vi "From Veristand Master To Modbus.vi"(7 "Parameters":T1 {"Interface Data"."Serial Settings"."parity (even)" items=["None", "Odd", "Even", "Mark", "Space"]; "Interface Data"."Serial Settings"."flow control (none)" items=["None", "XON/XOFF", "RTS/CTS", "XON/XOFF & RTS/CTS", "DTR/DSR", "XON/XOFF & DTR/DSR"]}, 8 "error in (no error)":errorcluster, 10 "Process in":refnum<class "Process.lvclass">, 11 "Modbus Master in":refnum<class "Modbus Master.lvclass">) -> ()   [LabVIEW 2015, in "Modbus Master Engine.lvlib"]
uses:
  Modbus Master Engine.lvlib
  <vilib>/addons/Inline Async API/_VS Inline Async API/Process/Process.lvclass
  Shared/Device Info.ctl
  Shared/Controls/Interface Type.ctl
  Shared/Controls/Data Model/TCP Settings.ctl
  Shared/Controls/Data Model/Serial Settings.ctl
  Bulk Data Access.ctl
  System Explorer/SubVIs/Modbus Type.ctl
  Shared/Controls/Data Model/Channel.ctl
  <vilib>/NI Veristand/Custom Device API/Custom Device Channel Type.ctl
  Shared/Controls/Data Model/Mapping.ctl
  Shared/Controls/Data Model/DataType.ctl
  <vilib>/NI Veristand/Custom Device API/Custom Device Item Ref.ctl
  Modbus API.lvlibp/API/Master/Modbus Master.lvclass
  <vilib>/addons/Inline Async API/_Data Access Engine/Access Type Classes/Read/Read.lvclass/Read.ctl
  <vilib>/addons/Inline Async API/_VS Inline Async API/Process/Process.lvclass/Process.ctl
  <vilib>/addons/Inline Async API/_Data Access Engine/Access Type Classes/Read/Read.ProcessData.vi
  <vilib>/addons/Inline Async API/_Data Access Engine/Data Access Engine/Methods/Read.Data.vi
  <vilib>/addons/Inline Async API/_Data Access Engine/Data Access Engine/Data Access Engine.lvclass
  Shared/Modbus Master Shared.lvlib
  <vilib>/NI VeriStand/Custom Device API/Custom Device API.lvlib
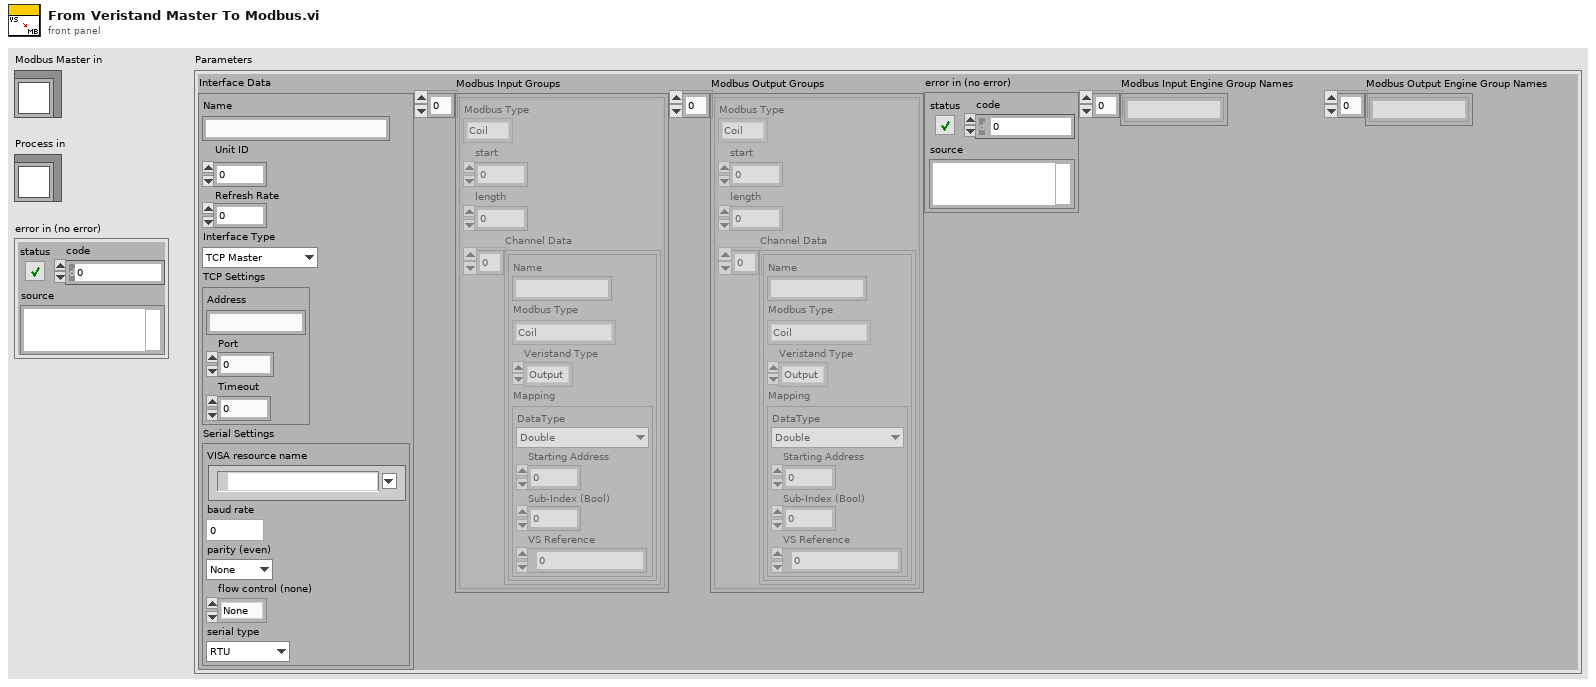
[diagram p1: front panel]
types:
  T1 = typedef "Modbus Master Shared.lvlib/Device Info.ctl" = cluster{"Interface Data":cluster{"Name":string, "Unit ID":u8, "Refresh Rate":i32, "Interface Type":T2, "TCP Settings":T3, "Serial Settings":T4}, "Modbus Input Groups":T5[], "Modbus Output Groups":T5[], "error in (no error)":errorcluster, "Modbus Input Engine Group Names":string[], "Modbus Output Engine Group Names":string[]}
  T2 = typedef "Modbus Master Shared.lvlib/Interface Type.ctl" = enum16{"TCP Master", "Serial Master", "TCP Slave", "Serial Slave"}
  T3 = typedef "Modbus Master Shared.lvlib/TCP Settings.ctl" = cluster{"Address":string, "Port":u16, "Timeout":i32}
  T4 = typedef "Modbus Master Shared.lvlib/Serial Settings.ctl" = cluster{"VISA resource name":refnum<visa-resource-name>, "baud rate":u32, "parity (even)":u16, "flow control (none)":u16, "serial type":enum16{"RTU", "ASCII"}}
  T5 = typedef "Modbus Master Shared.lvlib/Bulk Data Access.ctl" = cluster{"Modbus Type":T6, "start":u16, "length":u16, "Channel Data":T7[]}
  T6 = typedef "Modbus Master Shared.lvlib/Modbus Type.ctl" = enum16{"Coil", "Discrete Input", "Holding Register", "Input Register"}
  T7 = typedef "Modbus Master Shared.lvlib/Channel.ctl" = cluster{"Name":string, "Modbus Type":T6, "Veristand Type":T8, "Mapping":T9}
  T8 = typedef "Custom Device API.lvlib/Custom Device Channel Type.ctl" = enum16{"Input", "Output"}
  T9 = typedef "Modbus Master Shared.lvlib/Mapping.ctl" = cluster{"DataType":T10, "Starting Address":u16, "Sub-Index (Bool)":u16, "VS Reference":T11}
  T10 = typedef "Modbus Master Shared.lvlib/DataType.ctl" = enum16{"Double", "Single", "I64", "I32", "I16", "I8", "U64", "U32", "U16", "U8", "Boolean"}
  T11 = typedef "Custom Device API.lvlib/Custom Device Item Ref.ctl" = u64
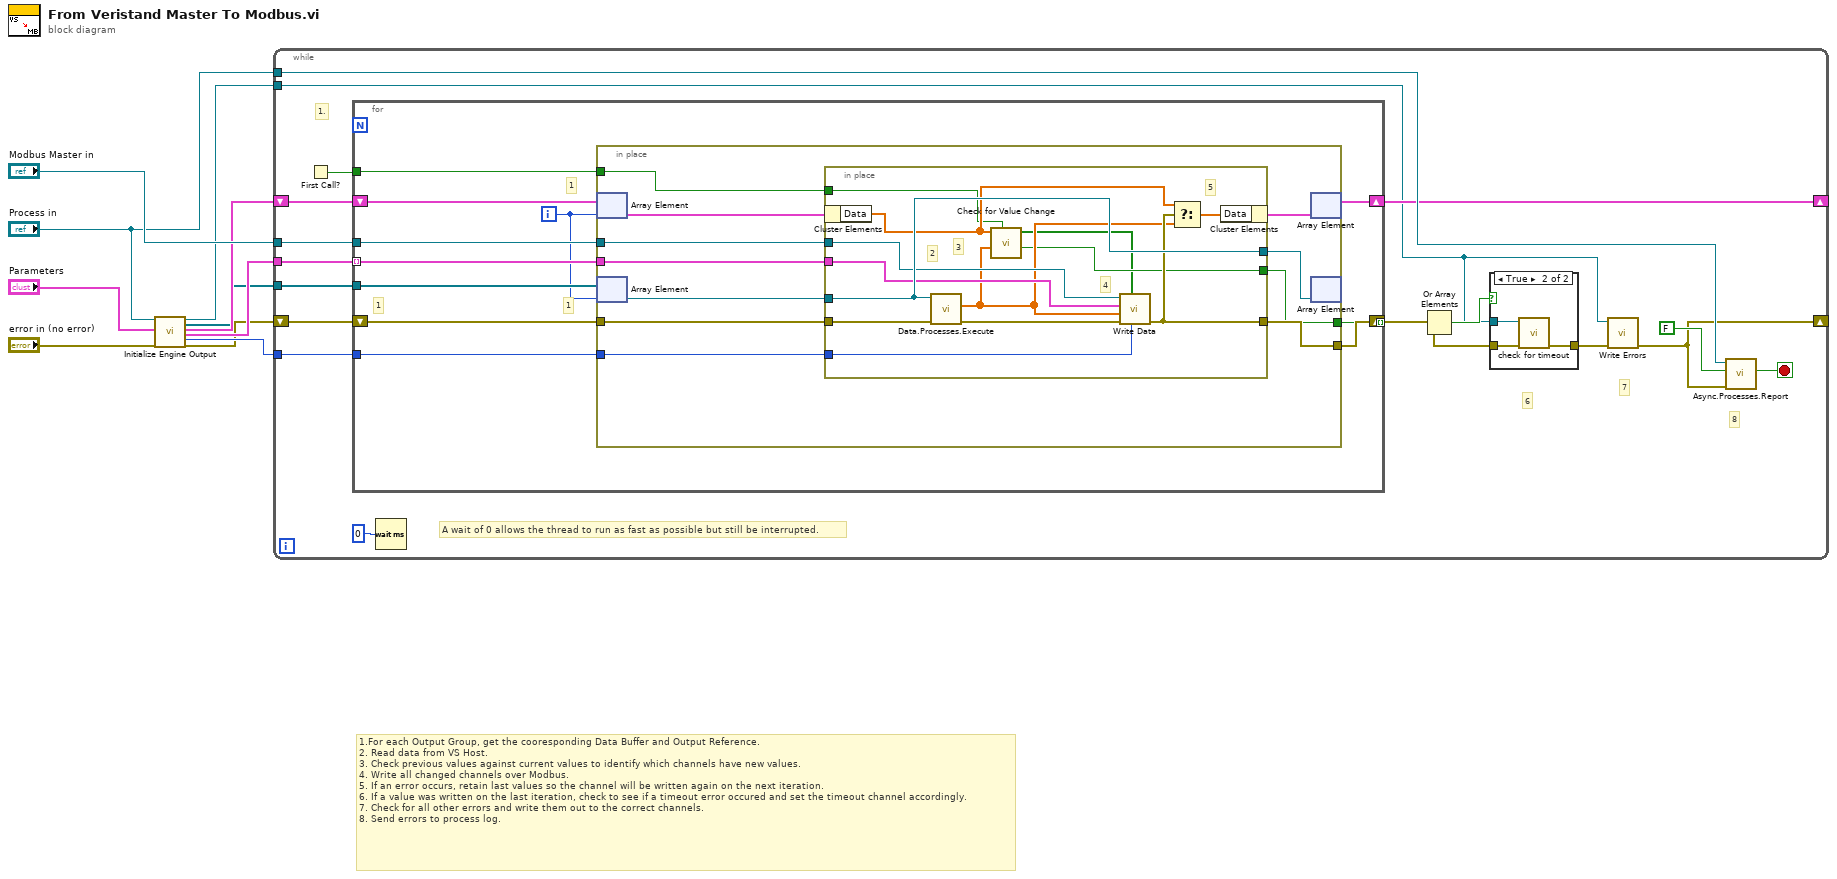
[diagram p0: block diagram]
diagram:
  # "1.For each Output Group, get the cooresponding Data Buffer and Output Reference.\n2. Read data from VS Host.\n3. Check previous values against current values to identify which channels have new values.\n4. Write all changed channels over Modbus.\n5. If an error occurs, retain last values so the channel will be written again on the next iteration.\n6. If a value was written on the last iteration, check to see if a timeout error occured and set the timeout channel accordingly.\n7. Check for all other errors and write them out to the correct channels.\n8. Send errors to process log."
  n1 = call "Initialize Engine Output.vi"("Process in"="Process in", "Parameters"="Parameters", "error in (no error)"="error in (no error)") -> ("Diagnostic Group Ref"=w3:refnum<data-value>, "Output Group Refs"=w5:refnum<data-value>[], "Data Buffers"=w7:cluster{"Data":dbl[]}[], "Modbus Output Groups"=w8:T5[], "Unit ID"=w2:u8, "error out"=w1:errorcluster)  [unwired: 11 in]
  n2 = while {
    tunnel: "Process in" -> [w28]
    tunnel: w5 -> [w25]
    tunnel: w8 -> [w27]
    tunnel: "Modbus Master in" -> [w26]
    shift-right: [w22] -> _
    shift-left: w7 -> [w23]
    tunnel: w3 -> [w11]
    tunnel: w2 -> [w18]
    shift-right: [w17] -> _
    shift-left: w1 -> [w16]
    stop <- w24 stop-if-true
    # "8"
    # "7"
    # "6"
    # "A wait of 0 allows the thread to run as fast as possible but still be interrupted."
    # "1."
    n3 = First Call?() -> (First Call?: T/F=w19:bool)
    n4 = for {
      tunnel: w27 -> [w38] mode=indexing
      tunnel: w26 -> [w39]
      tunnel: w25 -> [w34]
      shift-right: [w35] -> w22
      shift-left: w23 -> [w36]
      tunnel: w19 -> [w32]
      tunnel: w18 -> [w31]
      shift-right: [w30] -> w15
      shift-left: w16 -> [w37]
      tunnel: [w29] -> w13 mode=indexing
      i -> [w33]
      # "1"
      # "1"
      # "1"
      n5 = in-place {
        in-place-border: w39 -> [w50]
        in-place-border: w38 -> [w49]
        in-place-border: w37 -> [w48]
        in-place-border: [w47] -> w30
        in-place-border: w32 -> [w42]
        in-place-border: w31 -> [w41]
        in-place-border: [w40] -> w29
        n6 = in-place-array #1(w36, w33) -> (w46:cluster{"Data":dbl[]})
        n7 = in-place-array #2(w34, w33) -> (w44:refnum<data-value>)
        n8 = in-place {
          in-place-border: w50 -> [w61]
          in-place-border: w49 -> [w58]
          in-place-border: w48 -> [w62]
          in-place-border: [w57] -> w47
          in-place-border: w44 -> [w63]
          in-place-border: [w63] -> w43
          in-place-border: w42 -> [w51]
          in-place-border: w41 -> [w60]
          in-place-border: [w53] -> w40
          # "5"
          # "4"
          # "3"
          # "2"
          n9 = in-place-cluster #3(w46) -> ("Data"=w55:dbl[])
          n10 = call-poly <vilib>:"Data.Processes.Execute.vi"("error in (no error)"=w62, "Ref"=w63) -> ("error out"=w59:errorcluster, "Values"=w54:dbl[])  [unwired: 7 in, 1 out]
          n11 = call "Check for Value Change.vi"("Force Write?"=w51, "New Data"=w54, "Last Value Data"=w55) -> ("Value Change?"=w53:bool, "Indices to Update"=w52:bool[])  [unwired: 7 in]
          n12 = call "Write Data.vi"("Unit ID"=w60, "Write Mask"=w52, "error in (no error)"=w59, "Values"=w54, "output data access"=w58, "Modbus Master in"=w61) -> ("error out"=w57:errorcluster)  [unwired: 5 in]
          n13 = Select(t=w55, s=w57, f=w54) -> (s? t:f=w56:dbl[])
          n14 = in-place-cluster #3("Data"=w56) -> (w45:cluster{"Data":dbl[]})
        }
        n15 = in-place-array #1(w45) -> (w35:cluster{"Data":dbl[]}[])  [unwired: 1 out]
        n16 = in-place-array #2(w43) -> ()  [unwired: 2 out]
      }
    }
    n17 = Wait (ms)(milliseconds to wait=u32 0) -> ()  [unwired: 1 out]
    n18 = Or Array Elements(Boolean array=w13) -> (logical OR=w12:bool)
    n19 = case shown="True" w12 {
      tunnel: w15 -> [w64 w67]
      tunnel: [w64 w66] -> w14
      tunnel: w11 -> [_ w65]
      frame False {
      }
      frame True {
        n20 = call "check for timeout.vi"("error in (no error)"=w67, "Data Value Reference in"=w65) -> ("error out"=w66:errorcluster)  [unwired: 9 in]
      }
    }
    n21 = call "Write Errors.vi"("error in (no error)"=w14, "Data Value Reference in"=w11) -> ("error out"=w17:errorcluster)  [unwired: 9 in]
    n22 = call <vilib>:"Async.Processes.Report.vi"("Error"=w17, "Stop on Error?"=FALSE, "Process in"=w28) -> ("Stop"=w24:bool)  [unwired: 7 in, 1 out]
  }
